vi "ArithMeticOperation.vi"() -> ()   [LabVIEW 2020]
panel:
  out "QRESULT":dbl
  out "RRESULT":dbl
  in  "Q2":dbl
  in  "Quotient1":dbl
  out "DivideRESULT":dbl
  in  "Divide2":dbl
  in  "Divide1":dbl
  out "MultiRESULT":dbl
  in  "Multi2":dbl
  in  "Multi1":dbl
  out "SubRESULT":dbl
  in  "Sub 2":dbl
  in  "Sub1":dbl
  out "AddRESULT":dbl
  in  "AddOpperant 2":dbl
  in  "AddOpperant1":dbl
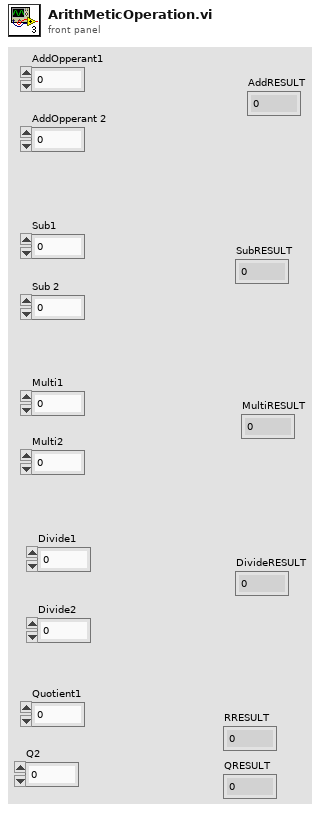
[diagram p1: front panel]
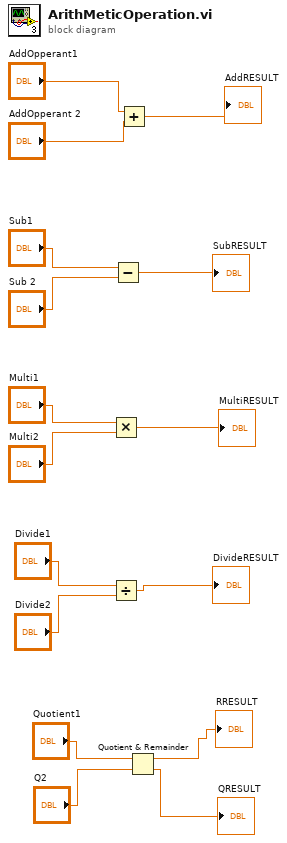
[diagram p0: block diagram]
diagram:
  n1 = Multiply(x="Multi1", y="Multi2") -> (x*y=→"MultiRESULT":dbl)
  n2 = Divide(x="Divide1", y="Divide2") -> (x/y=→"DivideRESULT":dbl)
  n3 = Subtract(x="Sub1", y="Sub 2") -> (x-y=→"SubRESULT":dbl)
  n4 = Add(x="AddOpperant1", y="AddOpperant 2") -> (x+y=→"AddRESULT":dbl)
  n5 = Quotient & Remainder(x="Quotient1", y="Q2") -> (x-y*floor(x/y)=→"RRESULT":dbl, floor(x/y)=→"QRESULT":dbl)
